vi "FTW-File-DereferenceNamespace.vi"(8 "error in":errorcluster, 11 "Base Filepath":path) -> (0 "error out":errorcluster, 2 "Actual Filepath":path)   [LabVIEW 2012]
panel:
  out "Regex Filter":string
  out "Matching Items":string[](array[string])
  # "Inputs"
  # "Debug"
  # "Outputs"
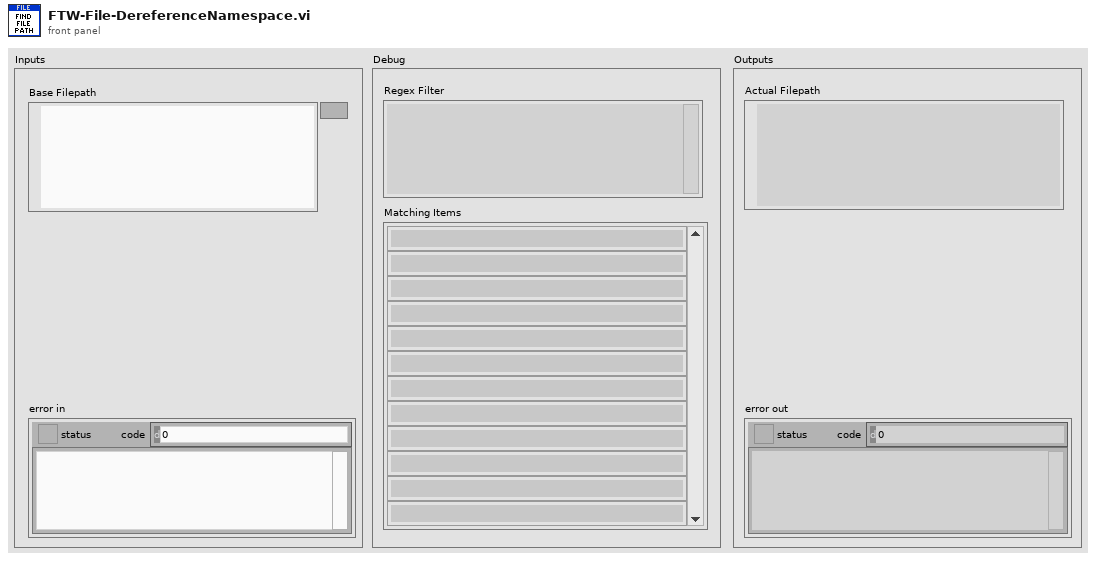
[diagram p1: front panel]
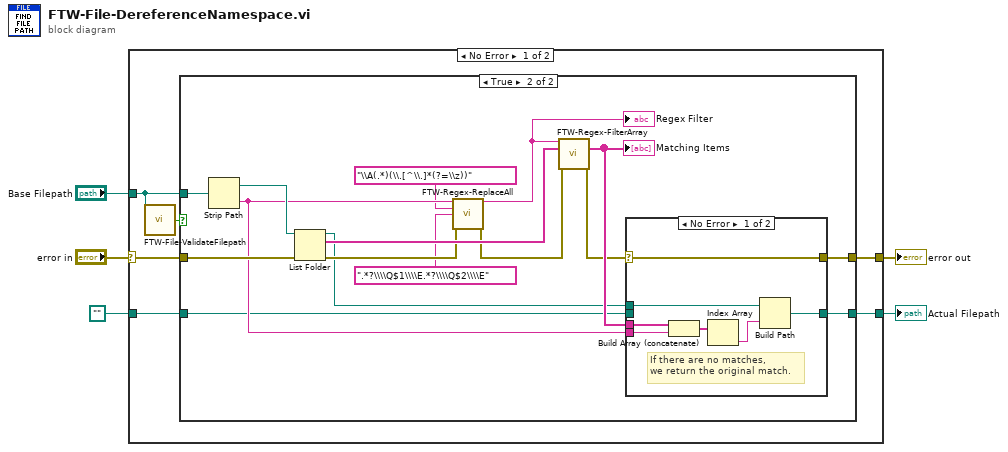
[diagram p0: block diagram]
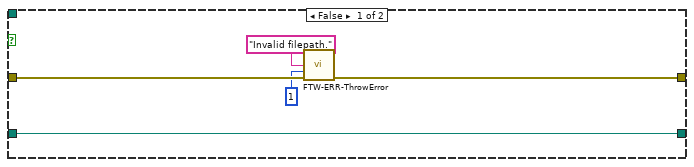
[diagram p2: hidden frame]
diagram:
  n1 = case shown="No Error" "error in" {
    selector: "error in" -> [w9 w43]
    tunnel: "Base Filepath" -> [w8 _]
    tunnel: [w11 w43] -> w4
    tunnel: [w7 w42] -> w2
    tunnel: path "" -> [w6 w42]
    frame No Error {
      n2 = call "FTW-File-ValidateFilepath.vi"("Filepath"=w8) -> ("Valid?"=w10:bool)
      n3 = case shown="True" w10 {
        tunnel: w9 -> [w16 w32]
        tunnel: [w15 w18] -> w11
        tunnel: w8 -> [_ w31]
        tunnel: [w12 w20] -> w7
        tunnel: w6 -> [w12 w17]
        frame False {
          n4 = call "FTW-ERR-ThrowError.vi"("Error Message"="Invalid filepath.", "Error Code"=1, "error in"=w16) -> ("error out"=w15:errorcluster)  [unwired: 12 in]
        }
        frame True {
          n5 = Strip Path(path=w31) -> (stripped path=w30:path, name=w27:string)
          n6 = List Folder(path=w30, error in=w32) -> (path out=w21:path, filenames=w29:string[], error out=w25:errorcluster)  [unwired: 3 out]
          n7 = call "FTW-Regex-ReplaceAll.vi"("String"=w27, "Search for (Regular Expression)"="\\A(.*)(\\.[^\\.]*(?=\\z))", "Replace with"=".*?\\\\Q$1\\\\E.*?\\\\Q$2\\\\E", "error in"=w25) -> ("String out"=w26:string, "error out"=w24:errorcluster)  [unwired: 9 in, 1 out]
          "Regex Filter" <- w26
          n8 = call "FTW-Regex-FilterArray.vi"("Regex Filter"=w26, "Input Array"=w29, "error in"=w24) -> ("Matching Items"=w28:string[], "error out"=w19:errorcluster)  [unwired: 10 in, 1 out]
          "Matching Items" <- w28
          n9 = case shown="No Error" w19 {
            selector: w19 -> [w33 w41]
            tunnel: w28 -> [w39 _]
            tunnel: w27 -> [w38 _]
            tunnel: w21 -> [w37 _]
            tunnel: [w36 w40] -> w20
            tunnel: [w33 w41] -> w18
            tunnel: w17 -> [_ w40]
            frame No Error {
              # "If there are no matches,\nwe return the original match."
              n10 = Build Array (concatenate)(w39, w38) -> (w35:string[])
              n11 = Index Array(array=w35) -> (element=w34:string)  [unwired: 1 in]
              n12 = Build Path(base path=w37, name or relative path=w34) -> (appended path=w36:path)
            }
            frame Error {
            }
          }
        }
      }
    }
    frame Error {
    }
  }
  "error out" <- w4
  "Actual Filepath" <- w2
